vi "Send TDC Arm Signal.vi"(8 "error in":errorcluster, 10 "master?":bool, 11 "FPGA VI Reference In":T1) -> (0 "error out":errorcluster, 3 "FPGA VI Reference Out":T1)   [LabVIEW 2011, in "FlexRIO Host Library (User).lvlib"]
uses:
  FlexRIO Host Library (User).lvlib
  Session/FPGA Session Ref.ctl
  <vilib>/rvi/interface/nirviReadWriteControl/nirviReadWriteControl.xnode
  Zeiss Acquisition Demo/FPGA Bitfiles/FlexRIODigitizer_FPGABoard_Acquire_Rev2.lvbitx
  <vilib>/rvi/errors/niLvFpgaMergeErrorWithErrorCode.vi
  <vilib>/rvi/errors/niLvFpgaAdjustHostInterfaceError.vi
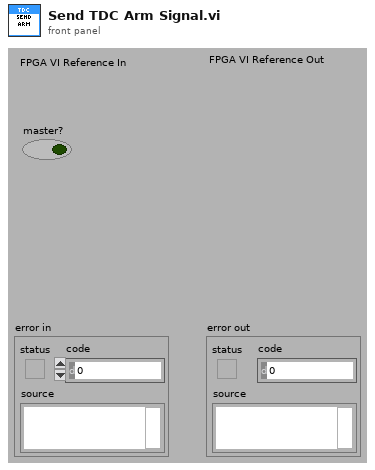
[diagram p1: front panel]
types:
  T1 = typedef "FlexRIO Host.lvlib/FPGA Session Ref.ctl" = refnum<k20>
  T2 = cluster{"clear meas valid":bool, "take a measurement":bool}
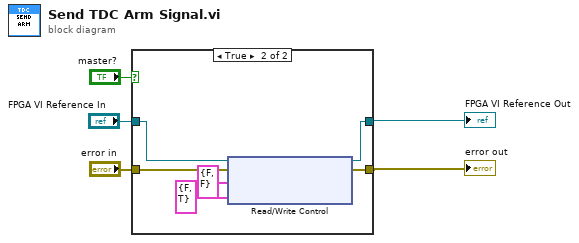
[diagram p0: block diagram]
diagram:
  n1 = case shown="True" "master?" {
    tunnel: "error in" -> [w6 w13]
    tunnel: "FPGA VI Reference In" -> [w7 w12]
    tunnel: [w6 w11] -> w1
    tunnel: [w7 w10] -> w2
    frame False {
    }
    frame True {
      n2 = xnode "Read/Write Control"("FPGA VI Reference In"=w12, "error in"=w13, "TDC Control Signals"=T2 {"clear meas valid"=FALSE, "take a measurement"=FALSE}, "TDC Control Signals"=T2 {"clear meas valid"=FALSE, "take a measurement"=TRUE}) -> ("FPGA VI Reference Out"=w10:T1, "error out"=w11:errorcluster)
    }
  }
  "error out" <- w1
  "FPGA VI Reference Out" <- w2
